vi "ConfigPanel.vi"(8 "error in (no error)":errorcluster, 11 "SEQ in":refnum<class "Sequence.lvclass">) -> (0 "error out":errorcluster, 3 "SEQ out":refnum<class "Sequence.lvclass">)   [LabVIEW 2012, in "StimulCtrls.lvlib"]
uses:
  StimulCtrls.lvlib
  UserControl/ElectdPanel.ctl
  UserControl/ElectdTerminal.ctl
  Sequence.lvclass
panel:
  in  "Stop Button":bool
  out "Tag":string
  in  "SEQ off":dbl[unit] format="%<%H:%M:%S%3u>t"
  in  "SEQ on":dbl[unit] format="%<%H:%M:%S%3u>t"
  out "SEQ Panel":T3 {"Electrode 16"."Magnitude" format="%4.2f"; "Electrode 15"."Magnitude" format="%4.2f"; "Electrode 14"."Magnitude" format="%4.2f"; "Electrode 13"."Magnitude" format="%4.2f"; "Electrode 12"."Magnitude" format="%4.2f"; "Electrode 11"."Magnitude" format="%4.2f"; "Electrode 10"."Magnitude" format="%4.2f"; "Electrode 9"."Magnitude" format="%4.2f"; "Electrode 8"."Magnitude" format="%4.2f"; "Electrode 7"."Magnitude" format="%4.2f"; "Electrode 6"."Magnitude" format="%4.2f"; "Electrode 5"."Magnitude" format="%4.2f"; "Electrode 4"."Magnitude" format="%4.2f"; "Electrode 3"."Magnitude" format="%4.2f"; "Electrode 2"."Magnitude" format="%4.2f"; "Electrode"."Magnitude" format="%4.2f"}
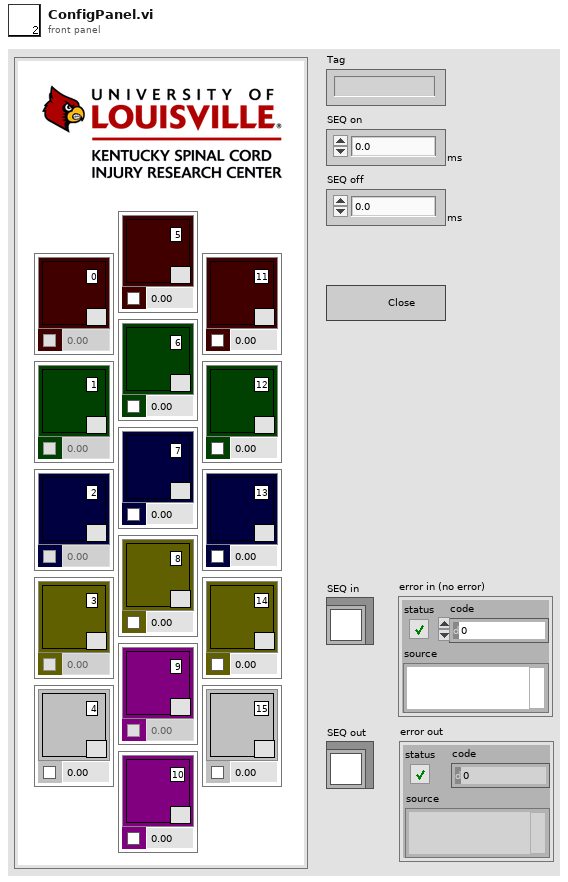
[diagram p1: front panel]
types:
  T1 = typedef "StimulCtrls.lvlib/ElectdPanel.ctl" = cluster{"Group #":string, "T #":T2, "Magnitude":sgl, "check":bool}
  T2 = typedef "StimulCtrls.lvlib/ElectdTerminal.ctl" = u8
  T3 = cluster{"Electrode":T1, "Electrode 2":T1, "Electrode 3":T1, "Electrode 4":T1, "Electrode 5":T1, "Electrode 6":T1, "Electrode 7":T1, "Electrode 8":T1, "Electrode 9":T1, "Electrode 10":T1, "Electrode 11":T1, "Electrode 12":T1, "Electrode 13":T1, "Electrode 14":T1, "Electrode 15":T1, "Electrode 16":T1}
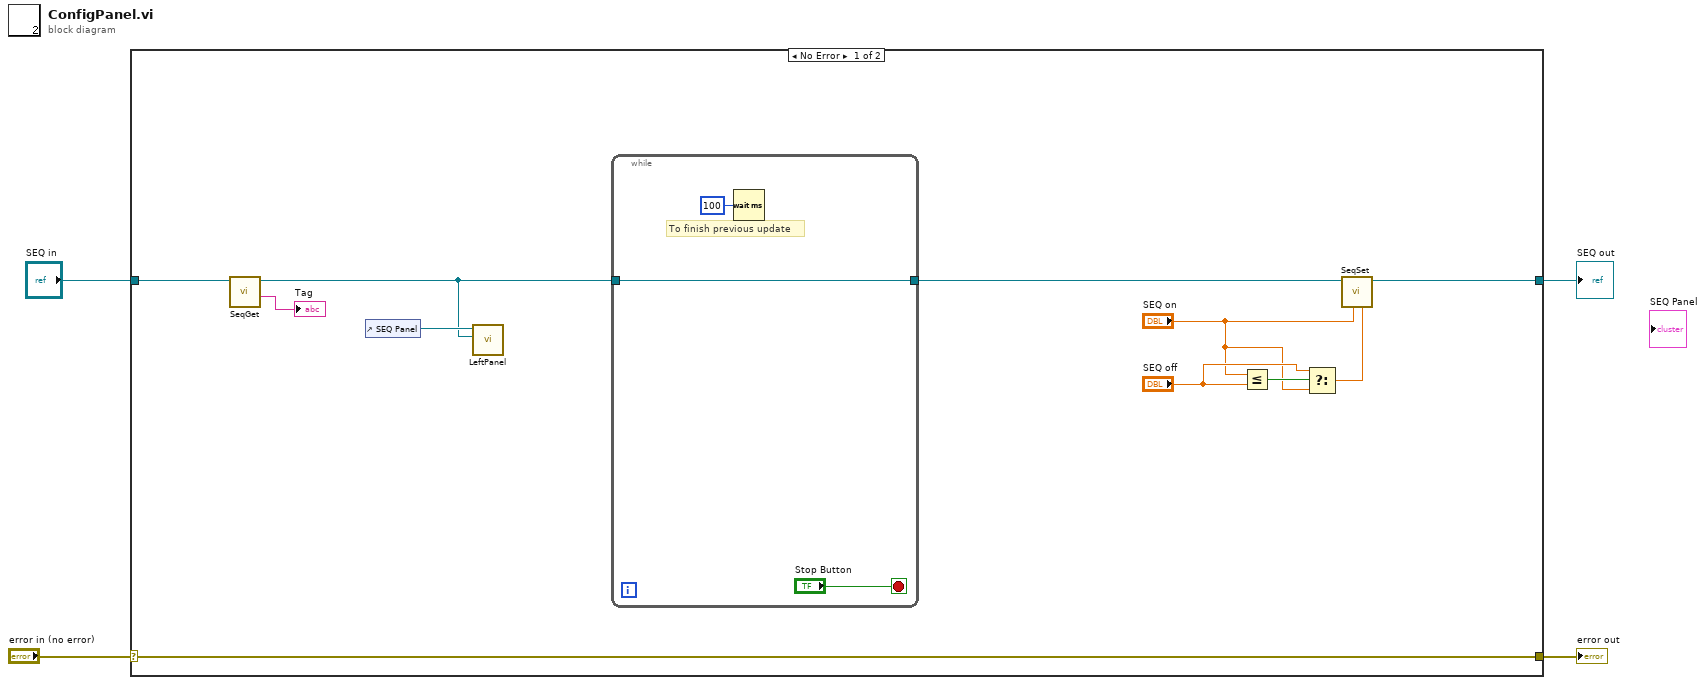
[diagram p0: block diagram]
diagram:
  n1 = case shown="No Error" "error in (no error)" {
    selector: "error in (no error)" -> [w15 w20]
    tunnel: [w15 w20] -> w3
    tunnel: [w10 w19] -> w2
    tunnel: "SEQ in" -> [w12 w19]
    frame No Error {
      n2 = call-dynamic "SeqGet.vi"("Sequence in"=w12) -> ("Tag"=→"Tag":string, "Sequence out"=w5:refnum<class "Sequence.lvclass">)  [unwired: 7 in, 2 out]
      n3 = control-ref of="SEQ Panel"() -> (w13:refnum<vi>)
      n4 = call "LeftPanel.vi"("Seqn in"=w5, "Panel Refnum"=w13) -> ()  [unwired: 9 in]
      n5 = while {
        tunnel: [w17] -> w11
        tunnel: w5 -> [w17]
        stop <- "Stop Button" stop-if-true
        # "To finish previous update"
        n6 = Wait (ms)(milliseconds to wait=u32 100) -> ()  [unwired: 1 out]
      }
      n7 = Less Or Equal?(x="SEQ on", y="SEQ off") -> (x <= y?=w9:bool)
      n8 = Select(t="SEQ off", s=w9, f="SEQ on") -> (s? t:f=w8:dbl[unit])
      n9 = call "SeqSet.vi"("Time off"=w8, "Time on"="SEQ on", "SEQ in"=w11) -> ("SEQ out"=w10:refnum<class "Sequence.lvclass">)  [unwired: 7 in, 1 out]
    }
    frame Error {
    }
  }
  "error out" <- w3
  "SEQ out" <- w2
